vi "ndipolaris Activate Wireless Tool.vi"(8 "error in (no error)":errorcluster, 9 "Location of ROM File for Tool":path, 11 "VISA resource name":refnum<visa-resource-name>) -> (0 "error out":errorcluster, 2 "Port Handle":string, 3 "VISA resource out":refnum<visa-resource-name>)   [LabVIEW 2013]
doc: "This VI assigns a port handle to a wireless tool. A ROM file that contains a description of the tool must be uploaded to the Polaris in order for the tool to be tracked. Creation of this file is not supported in LabVIEW. In order to create a ROM file, use the appropriate NDI software."
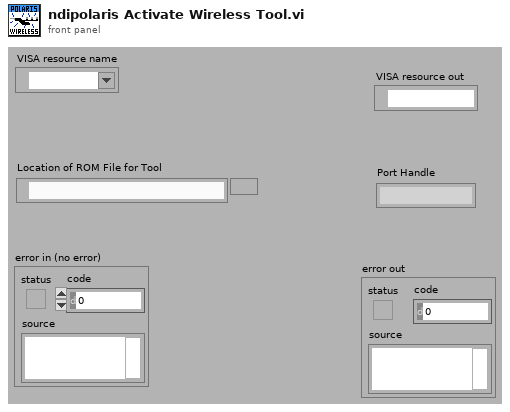
[diagram p1: front panel]
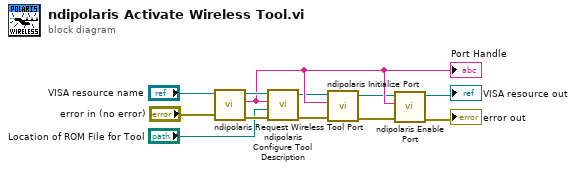
[diagram p0: block diagram]
diagram:
  n1 = call <instrlib>:"ndipolaris Request Wireless Tool Port.vi"("error in (no error)"="error in (no error)", "VISA resource name"="VISA resource name") -> ("error out"=w10:errorcluster, "Port Handle"=w7:string, "VISA resource out"=w9:refnum<visa-resource-name>)  [unwired: 7 in]
  "Port Handle" <- w7
  n2 = call <instrlib>:"ndipolaris Configure Tool Description.vi"("error in (no error)"=w10, "Location of ROM File for Tool"="Location of ROM File for Tool", "Port Handle"=w7, "VISA resource name"=w9) -> ("error out"=w4:errorcluster, "VISA resource out"=w5:refnum<visa-resource-name>)  [unwired: 6 in]
  n3 = call <instrlib>:"ndipolaris Initialize Port.vi"("error in (no error)"=w4, "Port Handle"=w7, "VISA resource name"=w5) -> ("error out"=w3:errorcluster, "VISA resource out"=w6:refnum<visa-resource-name>)  [unwired: 7 in]
  n4 = call <instrlib>:"ndipolaris Enable Port.vi"("error in (no error)"=w3, "Port Handle"=w7, "VISA resource name"=w6) -> ("error out"=→"error out":errorcluster, "VISA resource out"=→"VISA resource out":refnum<visa-resource-name>)  [unwired: 7 in]
